vi "Day 15-Find Valid Neighbors.vi"(10 "Current in":T1, 11 "Goal in":T1) -> (1 "All Neighbors":T1[](array[typedef]), 2 "Current out":T1, 3 "Goal out":T1)   [LabVIEW 2021]
uses:
  Day 15-Position.ctl
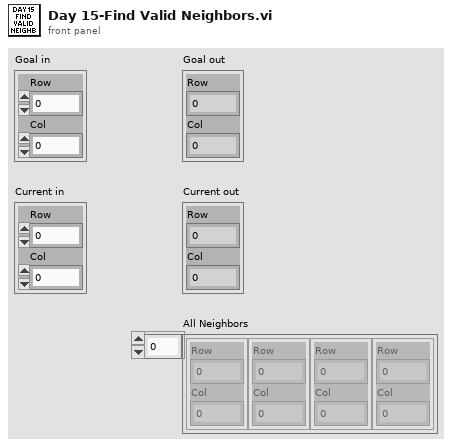
[diagram p1: front panel]
types:
  T1 = typedef "Day 15-Position.ctl" = cluster{"Row":i32, "Col":i32}
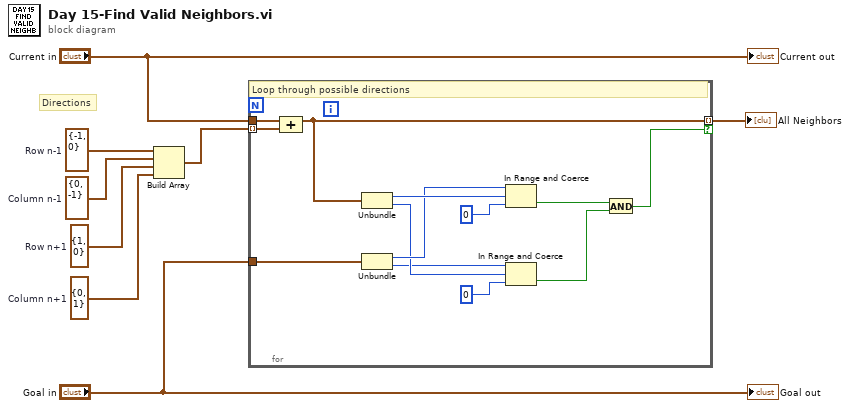
[diagram p0: block diagram]
diagram:
  w3 = T1 {"Row"=0, "Col"=1}  # Column n+1
  w4 = T1 {"Row"=1, "Col"=0}  # Row n+1
  w5 = T1 {"Row"=0, "Col"=-1}  # Column n-1
  w6 = T1 {"Row"=-1, "Col"=0}  # Row n-1
  # "Directions"
  n1 = Build Array(w6, w5, w4, w3) -> (w1:T1[])
  n2 = for {
    tunnel: "Current in" -> [w21]
    tunnel: [w18] -> w7 mode=indexing if=w9
    tunnel: "Goal in" -> [w20]
    tunnel: w1 -> [w19] mode=indexing
    # "Loop through possible directions"
    n3 = Compound Arithmetic op=ADD(w21, w19) -> (w18:T1)
    n4 = Unbundle(w18) -> ("Row"=w17:i32, "Col"=w14:i32)
    n5 = Unbundle(w20) -> ("Row"=w16:i32, "Col"=w13:i32)
    n6 = In Range and Coerce(upper limit=w16, x=w17, lower limit=0) -> (In Range?=w11:bool)  [unwired: 1 out]
    n7 = In Range and Coerce(upper limit=w13, x=w14, lower limit=0) -> (In Range?=w10:bool)  [unwired: 1 out]
    n8 = And(x=w11, y=w10) -> (x .and. y?=w9:bool)
  }
  "All Neighbors" <- w7
  "Current out" <- "Current in"
  "Goal out" <- "Goal in"
